vi "Read Waveform.vi"(8 "error in (no error)":errorcluster, 9 "Type":waveform(dbl), 10 "Tag":string, 11 "Var Bus in":refnum<class "Omni_Bus.lvclass">) -> (0 "error out":errorcluster, 2 "Waveform":waveform(dbl), 3 "Var Bus out":refnum<class "Omni_Bus.lvclass">)   [LabVIEW 2021, in "Omni_Bus.lvclass"]
uses:
  Omni_Bus.lvclass
  <vilib>/TSA/Abstract Data Classes/Abs_Types/Waveform/Abs_Waveform.lvclass
  C:/Program Files (x86)/National Instruments/LabVIEW 2021/vi.lib/TSA/Abstract Data Classes/Abs_Types/Type/Abs_Type.lvclass
  Omni_Bus.lvclass/Omni_Bus.ctl
  C:/Program Files (x86)/National Instruments/LabVIEW 2021/vi.lib/TSA/Abstract Data Classes/Abs_Types/Value/Abs_Value.lvclass
  C:/Program Files (x86)/National Instruments/LabVIEW 2021/vi.lib/TSA/Abstract Data Classes/Abs_Types/Collections/Vectors/Vector/Vector.lvclass
  C:/Program Files (x86)/National Instruments/LabVIEW 2021/vi.lib/TSA/Abstract Data Classes/Abs_Types/Iterator/Iterator.lvclass
  C:/Program Files (x86)/National Instruments/LabVIEW 2021/vi.lib/TSA/Abstract Data Classes/Abs_Types/Collections/Vectors/Vector_DBL/Vector_DBL.lvclass
  C:/Program Files (x86)/National Instruments/LabVIEW 2021/vi.lib/TSA/Abstract Data Classes/Abs_Types/Waveform/Abs_Waveform.lvclass
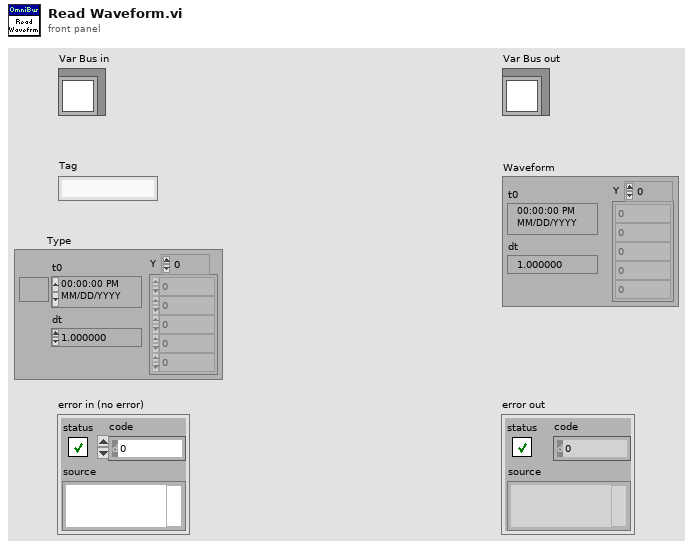
[diagram p1: front panel]
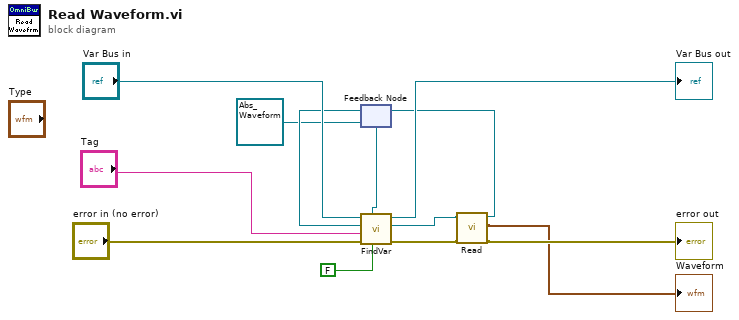
[diagram p0: block diagram]
diagram:
  w1 = refnum<class "Abs_Waveform.lvclass"> refnum ("Abs_Waveform out")
  n1 = feedback #1(w1) -> (w8:refnum<class "Abs_Waveform.lvclass">)
  n2 = call "FindVar.vi"("Write?"=FALSE, "Abs_Type"=w1, "error in (no error)"="error in (no error)", "Tag"="Tag", "Abs_Type Default"=w8, "Var Bus in"="Var Bus in") -> ("error out"=w7:errorcluster, "Abs_Type Found"=w6:refnum<class "Abs_Waveform.lvclass">, "Var Bus out"=→"Var Bus out":refnum<class "Omni_Bus.lvclass">)  [unwired: 2 in, 1 out]
  n3 = call-dynamic "Read.vi"("error in (no error)"=w7, "Abs_Waveform in"=w6) -> ("error out"=→"error out":errorcluster, "Waveform"=→"Waveform":waveform(dbl), "Abs_Waveform out"=w4:refnum<class "Abs_Waveform.lvclass">)  [unwired: 7 in]
  n4 = feedback-in #1(w4) -> ()
